vi "StringFunctions.TimeArrayToQueue.vi"(10 "Error In":errorcluster, 11 "TimeArray":refnum<data-value>) -> (2 "error out":errorcluster, 3 "queue out":refnum<queue>)   [LabVIEW 2016]
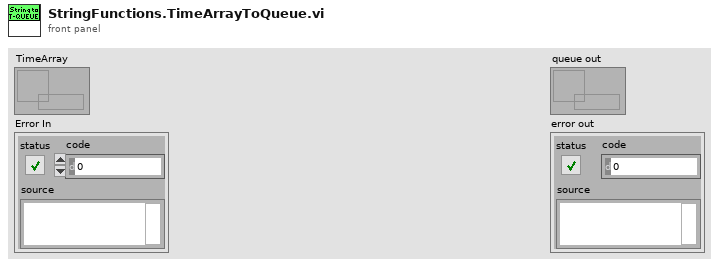
[diagram p1: front panel]
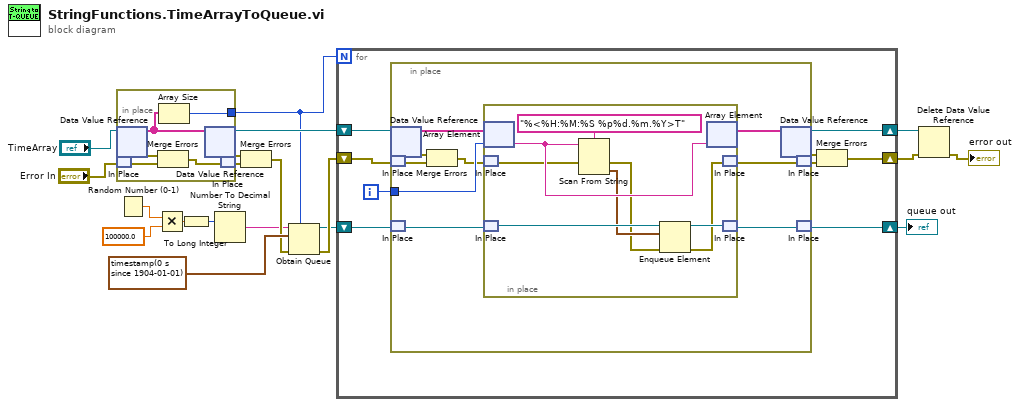
[diagram p0: block diagram]
diagram:
  n1 = in-place {
    in-place-border: [w21] -> w11
    n2 = in-place-dvr #1("TimeArray") -> (w20:string[], w24:errorcluster)
    n3 = in-place-match #2("Error In") -> (w23:errorcluster)
    n4 = Merge Errors(w24, w23) -> (w22:errorcluster)
    n5 = Array Size(array=w20) -> (size(s)=w21:i32)
    n6 = in-place-dvr #1(w20) -> (w15:refnum<data-value>, w17:errorcluster)
    n7 = in-place-match #2(w22) -> (w16:errorcluster)
  }
  n8 = Random Number (0-1)() -> (number: 0 to 1=w10:dbl)
  n9 = Multiply(x=w10, y=100000.0) -> (x*y=w8:dbl)
  n10 = To Long Integer(number=w8) -> (32bit integer=w7:i32)
  n11 = Number To Decimal String(number=w7) -> (decimal integer string=w6:string)  [unwired: 1 in]
  n12 = Merge Errors(w17, w16) -> (w13:errorcluster)
  n13 = Obtain Queue(max queue size (-1, unlimited)=w11, name (unnamed)=w6, element data type=timestamp(0 s since 1904-01-01), error in (no error)=w13) -> (queue out=w5:refnum<queue>, error out=w12:errorcluster)  [unwired: 1 in, 1 out]
  n14 = for {
    N: w11 -> [_]
    shift-right: [w32] -> w3
    shift-left: w15 -> [w33]
    shift-right: [w30] -> w1
    shift-left: w12 -> [w31]
    shift-right: [w25] -> w4
    shift-left: w5 -> [w26]
    i -> [w27]
    n15 = in-place {
      in-place-border: w27 -> [w38]
      n16 = in-place-dvr #3(w33) -> (w40:string[], w42:errorcluster)
      n17 = in-place-match #4(w31) -> (w41:errorcluster)
      n18 = in-place-match #5(w26) -> (w37:refnum<queue>)
      n19 = Merge Errors(w42, w41) -> (w35:errorcluster)
      n20 = in-place {
        n21 = in-place-array #6(w40, w38) -> (w47:string)
        n22 = in-place-match #7(w35) -> (w44:errorcluster)
        n23 = in-place-match #8(w37) -> (w49:refnum<queue>)
        n24 = Scan From String(format string="%<%H:%M:%S %p%d.%m.%Y>T", input string=w47, error in=w44) -> (error out=w43:errorcluster, output 1=w45:timestamp)  [unwired: 2 in, 2 out]
        n25 = Enqueue Element(queue=w49, element=w45, error in (no error)=w43) -> (queue out=w50:refnum<queue>, error out=w48:errorcluster)  [unwired: 1 in, 1 out]
        n26 = in-place-array #6(w47) -> (w39:string[])  [unwired: 1 out]
        n27 = in-place-match #7(w48) -> (w34:errorcluster)
        n28 = in-place-match #8(w50) -> (w36:refnum<queue>)
      }
      n29 = in-place-dvr #3(w39) -> (w32:refnum<data-value>, w28:errorcluster)
      n30 = in-place-match #4(w34) -> (w29:errorcluster)
      n31 = in-place-match #5(w36) -> (w25:refnum<queue>)
    }
    n32 = Merge Errors(w28, w29) -> (w30:errorcluster)
  }
  "queue out" <- w4
  n33 = Delete Data Value Reference(data value reference=w3, error in=w1) -> (error out=→"error out":errorcluster)  [unwired: 1 out]
